vi "TestBusClass.vi"() -> ()   [LabVIEW 2018, in "Bus.lvclass"]
uses:
  Bus.lvclass
  <userlib>/NIST/NISTErrorLib/NISTErrorLib.lvlib
panel:
  in  "ShowPanel? (f)":bool=TRUE
  in  "btnRemove":bool
  in  "Bus To Remove":i32
  in  "Bus To Add":i32
  in  "btnStop":bool
  in  "btnAdd":bool
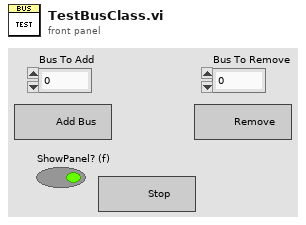
[diagram p1: front panel]
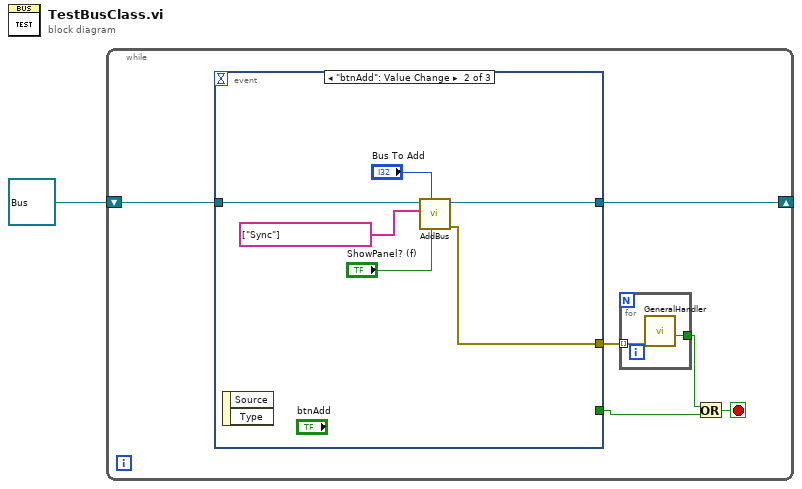
[diagram p0: block diagram]
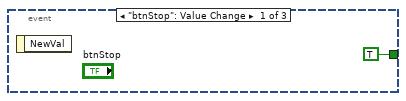
[diagram p2: hidden frame]
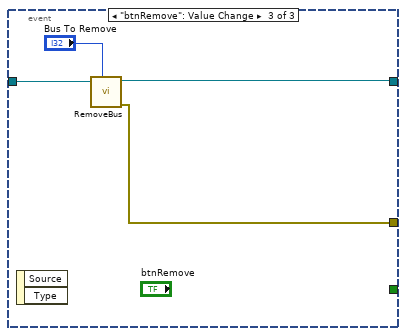
[diagram p3: hidden frame]
diagram:
  n1 = while {
    shift-right: [w6] -> _
    shift-left: refnum<class "Bus.lvclass"> refnum ("Bus.lvclass") -> [w7]
    stop <- w4 stop-if-true
    n2 = event shown="[1] \"btnAdd\": Value Change" {
      selector: _ -> [_ _ _]
      dyn-events: _ -> [_ _ _]
      timeout: _ -> [_ _ _]
      tunnel: [TRUE _ _] -> w3
      tunnel: w7 -> [_ w15 w20]
      tunnel: [_ w13 w17] -> w5
      tunnel: [_ w12 w19] -> w6
      event "btnStop": Value Change {
        n3 = event-data() -> ()  [unwired: 1 in, 1 out]
      }
      event "btnAdd": Value Change {
        n4 = event-data() -> ()  [unwired: 1 in, 2 out]
        n5 = call "AddBus.vi"("ShowPanel? (f)"="ShowPanel? (f)", "BusNumber"="Bus To Add", "ModuleList"=string[] ["Sync"], "Bus.lvclass"=w15) -> ("ErrorOut"=w13:errorcluster[], "Bus.lvclass"=w12:refnum<class "Bus.lvclass">)  [unwired: 5 in, 1 out]
      }
      event "btnRemove": Value Change {
        n6 = event-data() -> ()  [unwired: 1 in, 2 out]
        n7 = call "RemoveBus.vi"("BusNumber"="Bus To Remove", "Bus.lvclass"=w20) -> ("ErrorOut"=w17:errorcluster[], "Bus.lvclass"=w19:refnum<class "Bus.lvclass">)  [unwired: 8 in]
      }
    }
    n8 = for {
      tunnel: w5 -> [w9] mode=indexing
      tunnel: [w8] -> w2
      n9 = call <userlib>:"GeneralHandler.vi"("error in (no error)"=w9) -> ("Stop"=w8:bool)  [unwired: 7 in, 3 out]
    }
    n10 = Or(x=w2, y=w3) -> (x .or. y?=w4:bool)
  }
